vi "DSF.Engine.Framework.Get Transceiver Loader.vi"(11 "Framework in":refnum<class "DSF.Engine.Framework.lvclass">) -> (2 "Transceiver Loader":refnum<class "DSF.Engine.Transceiver Loader.lvclass">, 3 "Framework out":refnum<class "DSF.Engine.Framework.lvclass">)   [LabVIEW 2017, in "Data Sharing Framework Engine.lvlib" / "DSF.Engine.Framework.lvclass"]
uses:
  DSF.Engine.Framework.lvclass
  Transceiver/DSF.Engine.Transceiver Loader.lvclass
  DSF.Engine.Framework.lvclass/DSF.Engine.Framework.ctl
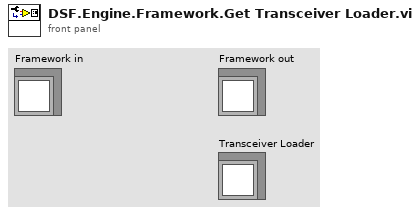
[diagram p1: front panel]
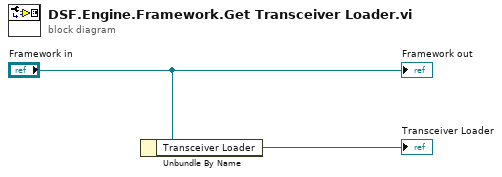
[diagram p0: block diagram]
diagram:
  n1 = Unbundle By Name("Framework in") -> ("Transceiver Loader"=→"Transceiver Loader":refnum<class "DSF.Engine.Transceiver Loader.lvclass">)
  "Framework out" <- "Framework in"
